vi "CFG Extract Array Info.vi"(0 "reference":refnum<vi>, 11 "error in":errorcluster) -> (4 "Value String":string, 6 "Delimiter(s)":string, 8 "Dimensions":i32, 10 "Element Type":T1, 15 "error out":errorcluster)   [LabVIEW 2017]
uses:
  Type Defs/CFG Tag Type Enum.ctl
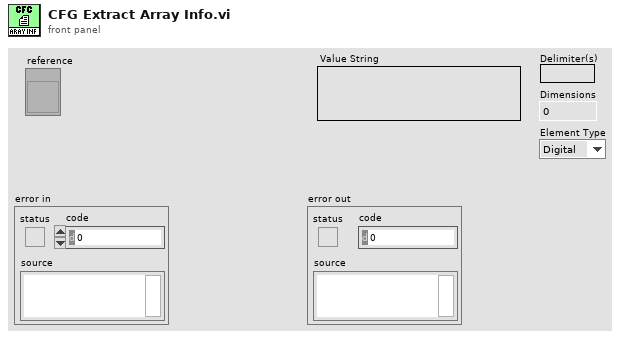
[diagram p1: front panel]
types:
  T1 = typedef "CFG Tag Type Enum.ctl" = enum16{"Digital", "Slide", "Enum", "Boolean", "String", "Path", "Array", "VISAResourceName", "DAQmxName", "Cluster"}
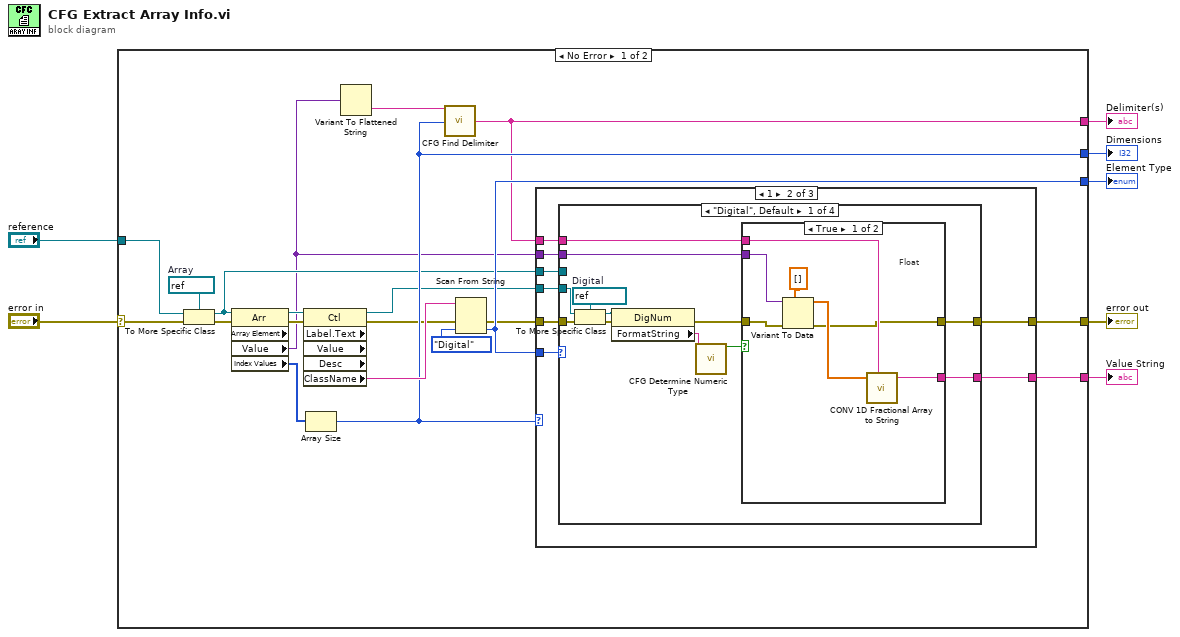
[diagram p0: block diagram]
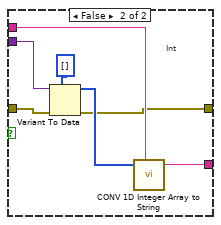
[diagram p3: hidden frame]
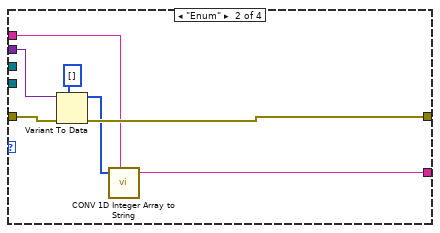
[diagram p4: hidden frame]
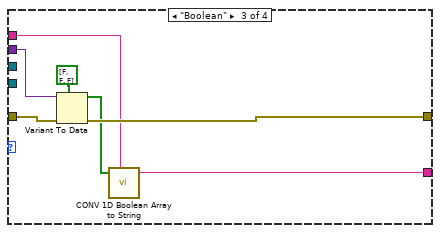
[diagram p5: hidden frame]
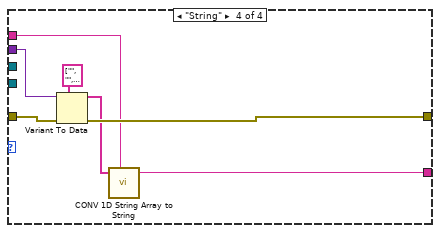
[diagram p6: hidden frame]
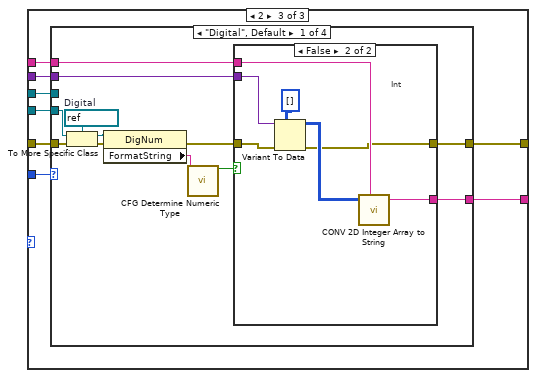
[diagram p7: hidden frame]
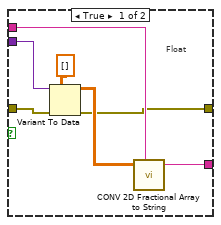
[diagram p8: hidden frame]
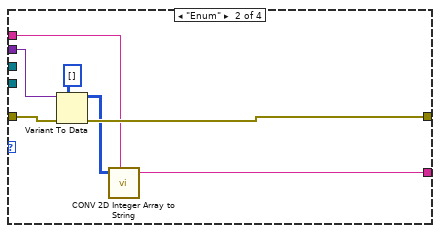
[diagram p9: hidden frame]
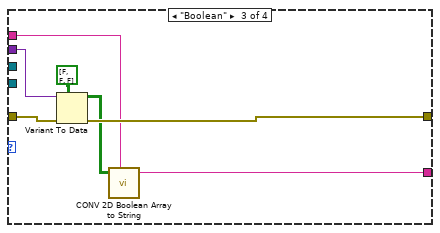
[diagram p10: hidden frame]
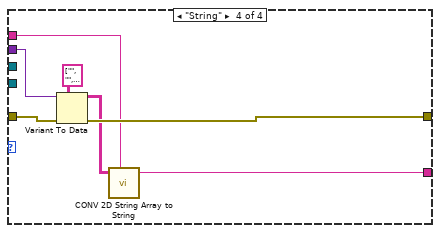
[diagram p11: hidden frame]
diagram:
  n1 = case shown="No Error" "error in" {
    selector: "error in" -> [w10 w139]
    tunnel: [w22 _] -> w7
    tunnel: [w21 _] -> w6
    tunnel: [w18 _] -> w5
    tunnel: [w17 _] -> w4
    tunnel: [w12 w139] -> w3
    tunnel: "reference" -> [w11 _]
    frame No Error {
      w27 = refnum<vi> refnum  # Array
      n2 = To More Specific Class(target class=w27, reference=w11, error in=w10) -> (specific class reference=w19:refnum<vi>, error out=w13:errorcluster)
      n3 = property class="Arr"(reference=w19, error in=w13) -> (error out=w14:errorcluster, "Array Element"=w26:refnum<vi>, "Value"=w8:variant, "Index Values"=w23:u32[])  [unwired: 1 out]
      n4 = property class="Ctl" props=["Label", "Text", "Value", "Desc", "ClassName"](reference=w26, error in=w14) -> (reference out=w20:refnum<vi>, error out=w15:errorcluster, "ClassName"=w25:string)  [unwired: 3 out]
      n5 = Array Size(array=w23) -> (size(s)=w22:i32)
      n6 = Variant To Flattened String(Variant=w8) -> (data string=w9:string)  [unwired: 1 out]
      n7 = call "CFG Find Delimiter.vi"("Value"=w9, "Dimensions"=w22) -> ("Delimiter (s)"=w18:string)  [unwired: 1 in, 12 out]
      n8 = Scan From String(input string=w25, error in=w15, default 1=CFG_Tag_Type_Enum."Digital" ("Type")) -> (error out=w16:errorcluster, output 1=w21:T1)  [unwired: 2 in, 2 out]
      n9 = case shown="1" w22 {
        tunnel: w21 -> [_ w36 w91]
        tunnel: w20 -> [_ w35 w90]
        tunnel: w19 -> [_ w34 w89]
        tunnel: w18 -> [_ w33 w88]
        tunnel: [_ w32 w87] -> w17
        tunnel: w8 -> [_ w31 w86]
        tunnel: [w28 w30 w85] -> w12
        tunnel: w16 -> [w28 w29 w84]
        frame Default {
        }
        frame 1 {
          n10 = case shown="\"Digital\", Default" w36 {
            tunnel: w35 -> [w47 _ _ _]
            tunnel: w34 -> [_ _ _ _]
            tunnel: w33 -> [w43 w64 w71 w78]
            tunnel: [w42 w69 w76 w83] -> w32
            tunnel: w31 -> [w37 w68 w75 w82]
            tunnel: [w38 w66 w73 w80] -> w30
            tunnel: w29 -> [w41 w63 w70 w77]
            frame "Digital", Default {
              w48 = refnum<vi> refnum  # Digital
              n11 = To More Specific Class(target class=w48, reference=w47, error in=w41) -> (specific class reference=w46:refnum<vi>, error out=w40:errorcluster)
              n12 = property class="DigNum"(reference=w46, error in=w40) -> (error out=w39:errorcluster, "FormatString"=w45:string)  [unwired: 1 out]
              n13 = call "CFG Determine Numeric Type.vi"("Format String"=w45) -> ("Float"=w44:bool)  [unwired: 14 out]
              n14 = case shown="True" w44 {
                tunnel: w43 -> [w54 w61]
                tunnel: [w55 w62] -> w42
                tunnel: w39 -> [w52 w59]
                tunnel: [w50 w57] -> w38
                tunnel: w37 -> [w49 w56]
                frame True {
                  # "Float"
                  n15 = Variant To Data(error in=w52, type=dbl[] [] ("1D Ring Array 2"), Variant=w49) -> (data=w51:dbl[], error out=w50:errorcluster)
                  n16 = call "CONV 1D Fractional Array to String.vi"("1-D Fractional"=w51, "Delimiter (,)"=w54) -> ("String"=w55:string)  [unwired: 2 in, 5 out]
                }
                frame False {
                  # "Int"
                  n17 = Variant To Data(error in=w59, type=i32[] [] ("1D Ring Array 2"), Variant=w56) -> (data=w58:i32[], error out=w57:errorcluster)
                  n18 = call "CONV 1D Integer Array to String.vi"("1-D Integer"=w58, "Delimiter (,)"=w61) -> ("String"=w62:string)  [unwired: 7 out]
                }
              }
            }
            frame "Enum" {
              n19 = Variant To Data(error in=w63, type=i32[] [] ("1D Ring Array 2"), Variant=w68) -> (data=w65:i32[], error out=w66:errorcluster)
              n20 = call "CONV 1D Integer Array to String.vi"("1-D Integer"=w65, "Delimiter (,)"=w64) -> ("String"=w69:string)  [unwired: 7 out]
            }
            frame "Boolean" {
              n21 = Variant To Data(error in=w70, type=bool[] [FALSE, FALSE, FALSE] ("1D Ring Array 2"), Variant=w75) -> (data=w72:bool[], error out=w73:errorcluster)
              n22 = call "CONV 1D Boolean Array to String.vi"("1-D Boolean"=w72, "Delimiter (,)"=w71) -> ("String"=w76:string)  [unwired: 1 in, 6 out]
            }
            frame "String" {
              n23 = Variant To Data(error in=w77, type=string[] ["", "", ""] ("1D Ring Array 2"), Variant=w82) -> (data=w79:string[], error out=w80:errorcluster)
              n24 = call "CONV 1D String Array to String.vi"("1-D String"=w79, "Delimiter (,)"=w78) -> ("String"=w83:string)  [unwired: 7 out]
            }
          }
        }
        frame 2 {
          n25 = case shown="\"Digital\", Default" w91 {
            tunnel: w90 -> [w102 _ _ _]
            tunnel: w89 -> [_ _ _ _]
            tunnel: w88 -> [w98 w119 w126 w133]
            tunnel: [w97 w124 w131 w138] -> w87
            tunnel: w86 -> [w92 w123 w130 w137]
            tunnel: [w93 w121 w128 w135] -> w85
            tunnel: w84 -> [w96 w118 w125 w132]
            frame "Digital", Default {
              w103 = refnum<vi> refnum  # Digital
              n26 = To More Specific Class(target class=w103, reference=w102, error in=w96) -> (specific class reference=w101:refnum<vi>, error out=w95:errorcluster)
              n27 = property class="DigNum"(reference=w101, error in=w95) -> (error out=w94:errorcluster, "FormatString"=w100:string)  [unwired: 1 out]
              n28 = call "CFG Determine Numeric Type.vi"("Format String"=w100) -> ("Float"=w99:bool)  [unwired: 14 out]
              n29 = case shown="False" w99 {
                tunnel: w98 -> [w109 w116]
                tunnel: [w110 w117] -> w97
                tunnel: w94 -> [w107 w114]
                tunnel: [w105 w112] -> w93
                tunnel: w92 -> [w104 w111]
                frame True {
                  # "Float"
                  n30 = Variant To Data(error in=w107, type=dbl[][] [] ("1D Ring Array 2"), Variant=w104) -> (data=w106:dbl[][], error out=w105:errorcluster)
                  n31 = call "CONV 2D Fractional Array to String.vi"("2-D Fractional"=w106, "Delimiters (,;)"=w109) -> ("String"=w110:string)  [unwired: 1 in, 6 out]
                }
                frame False {
                  # "Int"
                  n32 = Variant To Data(error in=w114, type=i32[][] [] ("1D Ring Array 2"), Variant=w111) -> (data=w113:i32[][], error out=w112:errorcluster)
                  n33 = call "CONV 2D Integer Array to String.vi"("2-D Integer"=w113, "Delimiters (,;)"=w116) -> ("String"=w117:string)  [unwired: 7 out]
                }
              }
            }
            frame "Enum" {
              n34 = Variant To Data(error in=w118, type=i32[][] [] ("1D Ring Array 2"), Variant=w123) -> (data=w120:i32[][], error out=w121:errorcluster)
              n35 = call "CONV 2D Integer Array to String.vi"("2-D Integer"=w120, "Delimiters (,;)"=w119) -> ("String"=w124:string)  [unwired: 7 out]
            }
            frame "Boolean" {
              n36 = Variant To Data(error in=w125, type=bool[][] [[FALSE, FALSE, FALSE]] ("1D Ring Array 2"), Variant=w130) -> (data=w127:bool[][], error out=w128:errorcluster)
              n37 = call "CONV 2D Boolean Array to String.vi"("2-D Boolean"=w127, "Delimiters (,;)"=w126) -> ("String"=w131:string)  [unwired: 1 in, 6 out]
            }
            frame "String" {
              n38 = Variant To Data(error in=w132, type=string[][] [["", "", ""]] ("1D Ring Array 2"), Variant=w137) -> (data=w134:string[][], error out=w135:errorcluster)
              n39 = call "CONV 2D String Array to String.vi"("2-D String"=w134, "Delimiters (,;)"=w133) -> ("String"=w138:string)  [unwired: 7 out]
            }
          }
        }
      }
    }
    frame Error {
    }
  }
  "Delimiter(s)" <- w5
  "Dimensions" <- w7
  "Element Type" <- w6
  "Value String" <- w4
  "error out" <- w3
